vi "Create Semaphore(8.5).vi"(4 "error in (no error)":errorcluster, 5 "return existing (F)":bool, 6 "size (1)":i32=1, 7 "name (unnamed)":string) -> (0 "error out":errorcluster, 1 "created new":bool, 3 "semaphore":T1)   [LabVIEW 2014]
doc: "LabVIEW no longer supports this VI. Use the Obtain Semaphore Reference VI instead. However, the Embedded Module for ARM Microcontrollers, Embedded Module for Blackfin Processors, Microprocessor SDK, Touch Panel Module, and Windows Mobile Module still support this VI.\n\nLooks up an existing semaphore or creates a new semaphore and returns a refnum. You can use this refnum when calling other Semaphore VIs.\n\n<B>Note</B> You cannot use semaphores to communicate between LabVIEW application instances. If you create a semaphore reference in one application instance, you cannot use that semaphore reference in another application instance."
uses:
  <vilib>/Utility/semaphor.llb/Semaphore Name & Ref DB Action.ctl
panel:
  in  "warning":errorcluster={"status"=FALSE, "code"=42, "source"="<err>User requested a named semaphore of a given size. The existing semaphore of that name had a different size. The existing semaphore was returned, size unchanged."}
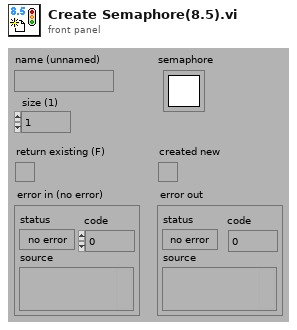
[diagram p1: front panel]
types:
  T1 = typedef "Semaphore RefNum" = refnum<k1>
  T2 = typedef "Semaphore Name & Ref DB Action.ctl" = enum16{"Lookup", "Insert", "Remove"}
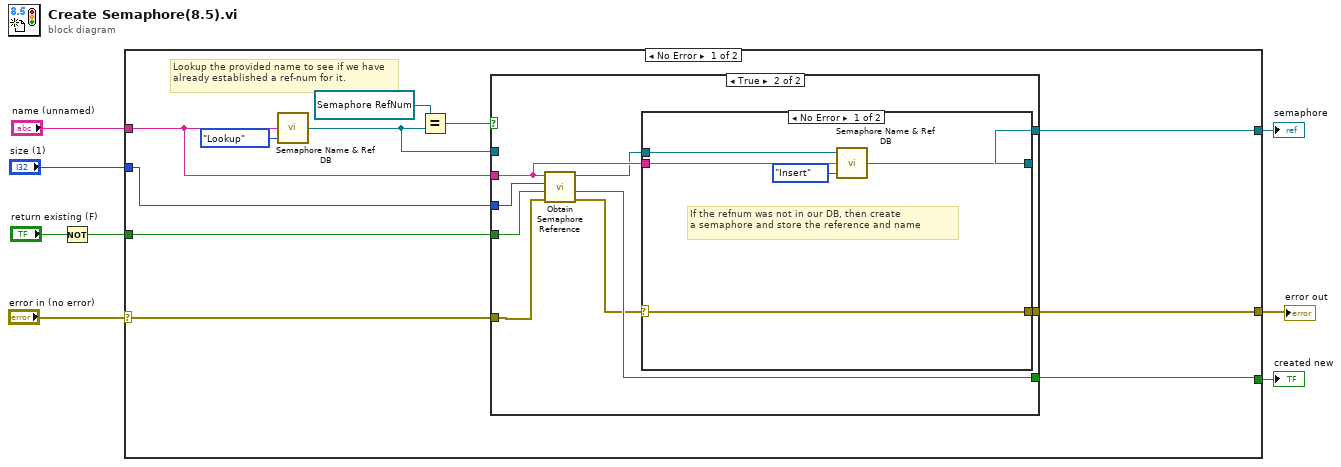
[diagram p0: block diagram]
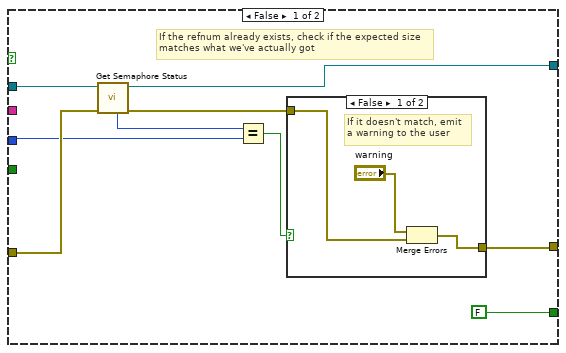
[diagram p2: hidden frame]
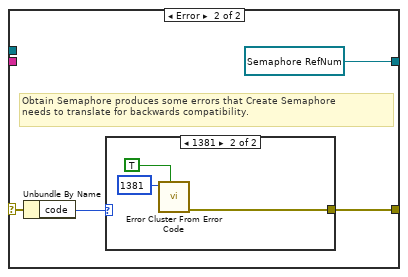
[diagram p4: hidden frame]
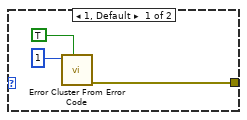
[diagram p5: hidden frame]
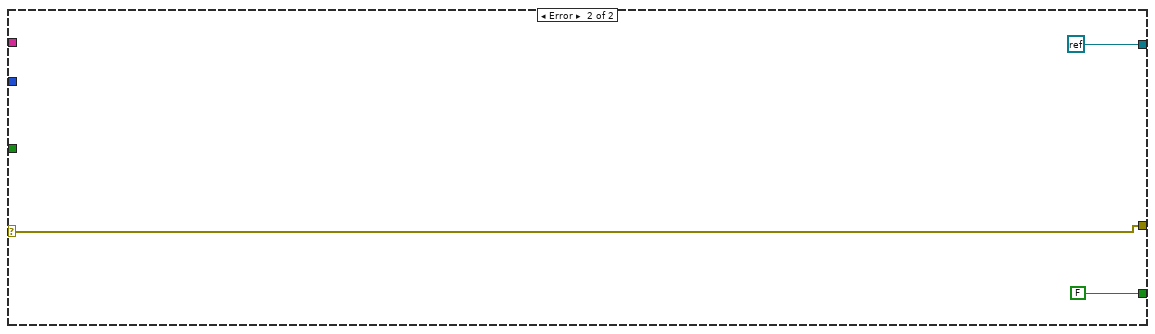
[diagram p6: hidden frame]
diagram:
  n1 = Not(x="return existing (F)") -> (.not. x?=w1:bool)
  n2 = case shown="No Error" "error in (no error)" {
    selector: "error in (no error)" -> [w16 w57]
    tunnel: w1 -> [w10 _]
    tunnel: "name (unnamed)" -> [w11 _]
    tunnel: [w12 refnum<k0> refnum] -> w7
    tunnel: [w14 FALSE ("created new?")] -> w6
    tunnel: "size (1)" -> [w15 _]
    tunnel: [w13 w57] -> w3
    frame No Error {
      w9 = T1 refnum items=["semaphore"] ("x")
      # "Lookup the provided name to see if we have already established a ref-num for it."
      n3 = call <vilib>:"Semaphore Name & Ref DB.vi"("Semaphore Action"=Semaphore_Name_&_Ref_DB_Action."Lookup", "Semaphore Name"=w11) -> ("semaphore ref out"=w17:T1)  [unwired: 1 in]
      n4 = Equal?(x=w9, y=w17) -> (x = y?=w18:bool)
      n5 = case shown="True" w18 {
        tunnel: w17 -> [w28 _]
        tunnel: w16 -> [w27 w39]
        tunnel: w15 -> [w25 w41]
        tunnel: [w22 w36] -> w13
        tunnel: [FALSE w38] -> w14
        tunnel: [w20 w33] -> w12
        tunnel: w11 -> [_ w35]
        tunnel: w10 -> [_ w40]
        frame False {
          # "If the refnum already exists, check if the expected size matches what we've actually got"
          n6 = call <vilib>:"Get Semaphore Status.vi"("error in (no error)"=w27, "semaphore"=w28) -> ("error out"=w23:errorcluster, "semaphore out"=w20:T1, "size"=w26:i32)  [unwired: 7 out]
          n7 = Equal?(x=w26, y=w25) -> (x = y?=w24:bool)
          n8 = case shown="False" w24 {
            tunnel: w23 -> [w31 w32]
            tunnel: [w29 w32] -> w22
            frame False {
              # "If it doesn't match, emit a warning to the user"
              n9 = Merge Errors("warning", w31) -> (w29:errorcluster)
            }
            frame True {
              # "If it does match, don't\nmodify the error wire"
            }
          }
        }
        frame True {
          n10 = call <vilib>:"Obtain Semaphore Reference.vi"("error in (no error)"=w39, "create if not found (T)"=w40, "size (1)"=w41, "name (unnamed)"=w35) -> ("error out"=w37:errorcluster, "created new"=w38:bool, "semaphore"=w34:T1)  [unwired: 1 in]
          n11 = case shown="No Error" w37 {
            selector: w37 -> [w46 w48]
            tunnel: [w46 w50] -> w36
            tunnel: w35 -> [w44 _]
            tunnel: w34 -> [w43 _]
            tunnel: [w42 w47] -> w33
            frame No Error {
              # "If the refnum was not in our DB, then create \na semaphore and store the reference and name"
              n12 = call <vilib>:"Semaphore Name & Ref DB.vi"("Semaphore Action"=Semaphore_Name_&_Ref_DB_Action."Insert", "Semaphore Name"=w44, "semaphore ref in"=w43) -> ("semaphore ref out"=w42:T1)
            }
            frame Error {
              w47 = T1 refnum items=["semaphore"] ("semaphore ref out")
              # "Obtain Semaphore produces some errors that Create Semaphore \nneeds to translate for backwards compatibility."
              n13 = Unbundle By Name(w48) -> ("code"=w49:i32)
              n14 = case shown="1381" w49 {
                tunnel: [w51 w54] -> w50
                frame 1, Default {
                  n15 = call <vilib>:"Error Cluster From Error Code.vi"("show call chain? (False)"=TRUE, "error code (0)"=1) -> ("error out"=w51:errorcluster)  [unwired: 1 in, 6 out]
                }
                frame 1381 {
                  n16 = call <vilib>:"Error Cluster From Error Code.vi"("show call chain? (False)"=TRUE, "error code (0)"=1381) -> ("error out"=w54:errorcluster)  [unwired: 1 in, 6 out]
                }
              }
            }
          }
        }
      }
    }
    frame Error {
    }
  }
  "error out" <- w3
  "semaphore" <- w7
  "created new" <- w6
